vi "CSV Log Loop.vi"(8 "error in (no error)":errorcluster, 11 "Message Queues":T65) -> (0 "error out":errorcluster)   [LabVIEW 2018, in "CSV Log.lvlib"]
uses:
  CSV Log.lvlib
  Main/Main Queue Cluster.ctl
  support/Message Queue/Message Cluster.ctl
  Drag and Drop/State Cluster.ctl
  Drag and Drop/Thumbnail Cluster.ctl
  Drag and Drop/Object Cluster.ctl
  <vilib>/Utility/miscctls.llb/LVRectTypeDef.ctl
  Drag and Drop/Object Type Enum.ctl
  <vilib>/Utility/miscctls.llb/LVPositionTypeDef.ctl
  Config Module/Controls/Main Config Cluster.ctl
  OPC/OPC Module Config.ctl
  Scale Module Folder/Measure Instrument/State Enum.ctl
  <vilib>/Utility/miscctls.llb/LVPoint32TypeDef.ctl
  OPC/OPC Settings.ctl
  OPC/Variable Data Cluster.ctl
  <vilib>/OPCUA/controls/NodeId.ctl
  <vilib>/OPCUA/controls/OPC UA StatusCode.ctl
  <vilib>/OPCUA/controls/Subscription ID.ctl
  <vilib>/OPCUA/controls/OPC UA Client Refnum.ctl
  <vilib>/OPCUA/controls/Subscription Data Change.ctl
  <vilib>/OPCUA/controls/Data Type.ctl
  Feed Module/Controls/Feed Module Config Cluster.ctl
  Feed Module/Controls/Feed Module Settings Cluster.ctl
  Ismatec ISM 831C/Controls/Ismatech Settings Cluster.ctl
  Masterflex 7550-30/Controls/Settings Cluster.ctl
  Mettler Toledo/Controls/Settings Cluster.ctl
  Bronkhorst M13 Flow Meter/Settings Cluster.ctl
  Measure Instrument/PID 2 Parameters Cluster.ctl
  Measure Instrument/PID Input Enum.ctl
  Measure Instrument/PID 2 Output Enum.ctl
  Tacmina QI/Tacmina QI DAQ Setting.ctl
  KNF Pump/Settings Cluster plus SIMDOS.ctl
  ASIA Pump/Pump Settings.ctl
  VICI M50 Party Mode/Settings Cluster.ctl
  FLOM Pump/Settings Cluster.ctl
  SSI PR Class/SSI PR or LD Settings Cluster.ctl
  Masterflex 75211/Masterflex 75211 DAQ Setting.ctl
  SSI PR Class/SSI P40 Settings Cluster.ctl
  TT Module/Controls/TT Module Config Cluster.ctl
  Tag VIs/Numeric Alarm Settings Cluster.ctl
  Acquisition/Hardware Configuration.ctl
  Acquisition/Task Cluster.ctl
  PT Module/Controls/PT Module Config Cluster.ctl
  Scale Module Folder/Feed Module/Controls/Scale Module Config Cluster.ctl
  Scale Module Folder/Feed Module/Controls/Scale Module Settings Cluster.ctl
  Pump Module Folder/Pump Module Config Cluster.ctl
  Pump Module Folder/Pump Module Settings Cluster.ctl
  LabJack Module/Controls/U3 Module Config Cluster.ctl
  Decoration Module/Decoration Module Config Cluster.ctl
  Flow Module Folder/Feed Module/Controls/Flow Module Config Cluster.ctl
  Flow Module Folder/Feed Module/Controls/Flow Module Settings Cluster.ctl
  TCU Module/TCU Module Folder/TCU Module Config Cluster.ctl
  TCU Module/TCU Module Folder/TCU Module Settings Cluster.ctl
  TCU Module/TCU Module Folder/Measure Instrument/Output Devices.ctl
  Huber TCU/Huber Settings.ctl
  Lauda Integral XT-150 TCU/Lauda Settings.ctl
  Julabo Type 1 TCU/Julabo Type 1 TCU Folder/Julabo FP-50 Settings.ctl
  Huber Unistat 410 TCU/Huber Unistat 410 RS485 Settings.ctl
  D-O Module Folder/Not Sure Where this is Used.ctl
  Sequencing/Squence Control.ctl
  D-O Module Folder/D-O Module Config Cluster.ctl
  D-O Module Folder/Valve Clusters.ctl
  D-O Module Folder/D-O Module Settings Cluster.ctl
  D-O Module Folder/D-O Device Settings Cluster.ctl
  VICI Electronic Actuator/VICI Electronic Actuator Settings.ctl
  Pressure Regulator Control Module/Pressure Regulator/Controls/4-20mA Module Config Cluster.ctl
  Pressure Regulator Control Module/Pressure Regulator/Controls/4-20mA Module Settings Cluster.ctl
  Pressure Transmitter/Pressure Transmitter Device Settings.ctl
  Pressure Reg Module/Pressure Regulator Device Settings.ctl
  CSV Log State Cluster.ctl
  support/Message Queue/Enqueue Message (Single).vi
  support/Message Queue/Message Queue.lvlib
  support/Command Log VIs/Command Logging.lvlib
  TT Module/TT Module.lvlib
  Ismatec ISM 831C/Ismatec ISM 831C.lvlib
  Masterflex 7550-30/Masterflex 7550-30.lvlib
  Mettler Toledo/Mettler Toledo.lvlib
  Bronkhorst M13 Flow Meter/Bronkhorst M13 Flow Meter.lvlib
  Tacmina QI/Tacmina QI.lvlib
  KNF Pump/KNF SIMDOS.lvlib
  ASIA Pump.lvlib
  VICI M50 Party Mode/VICI M6 M50 Party Mode.lvlib
  Feed Module/Feed Module.lvlib
  DAQ/DAQ.lvlib
  PT Module/PT Module.lvlib
  Scale Module Folder/Scale Module.lvlib
  Pump Module Folder/Pump Module.lvlib
  LabJack Module/U3 Module.lvlib
  Flow Module Folder/Flow Module.lvlib
  Huber TCU/Huber Ministat 230 TCU.lvlib
  Lauda Integral XT-150 TCU/Lauda TCU.lvlib
  Julabo Type 1 TCU/Julabo Type 1 TCU Folder/Julabo Type FP-50 TCU.lvlib
  TCU Module/TCU Module Folder/TCU Module.lvlib
  Sequencing/Sequencing Library.lvlib
  D-O Module Folder/D-O Module.lvlib
  Config Module/Config Module.lvlib
  Drag and Drop/Drag and Drop.lvlib
  Pressure Transmitter/Pressure Transmitter Library.lvlib
  Pressure Regulator Control Module/Pressure Regulator/4-20mA Module.lvlib
  Pressure Reg Module/Pressure Regulator Library.lvlib
  FLOM Pump/FLOM Pump.lvlib
  SSI PR Class/SSI PR or LD Pump.lvlib
  OPC/OPC UA.lvlib
  Scale Module Folder/Measure Instrument/Scale Module Engine.lvlib
  D-O Module Folder/DIO Valve/VICI Electronic Actuator.lvlib
  Masterflex 75211/Masterflex 75211.lvlib
  SSI PR Class/SSI P40 Pump.lvlib
  Huber Unistat 410 TCU/Huber Unistat 410 TCU.lvlib
panel:
  in  "?":T1 {"Main Config"."PR Module Configs"."Settings"."PID 2 Parameters"."output range"."output low" format="%.2f"; "Main Config"."PR Module Configs"."Settings"."PID 2 Parameters"."output range"."output high" min=0.0 max=100.0 format="%.2f"; "Main Config"."PR Module Configs"."Settings"."PID 2 Parameters"."PID gains"."derivative time (Td, min)" format="%.3f"; "Main Config"."PR Module Configs"."Settings"."PID 2 Parameters"."PID gains"."integral time (Ti, min)" format="%.3f"; "Main Config"."PR Module Configs"."Settings"."PID 2 Parameters"."PID gains"."proportional gain (Kc)" format="%.3f"; "Main Config"."Steps"."Control" items=["Pump %", "Setpoint"]; "Main Config"."TCU Module Configs"."Settings"."Huber Unistat 410 Settings"."Address" min=0 max=99 format="%02.0f"; "Main Config"."TCU Module Configs"."Settings"."Julabo FP-50 Settings"."Pump Power" min=0 max=8 step=1; "Main Config"."TCU Module Configs"."Settings"."Lauda Settings"."Pump Power" min=0 max=8 step=1; "Main Config"."Pump Module Configs"."Settings"."ASIA Pump C"."channel" min=0 max=1 step=1; "Main Config"."Pump Module Configs"."Settings"."Masterflex"."Pump Number" min=1.0 max=20.0 step=1.0; "Main Config"."Pump Module Configs"."Settings"."Ismatech"."Pump Number" min=1.0 max=20.0 step=1.0; "Main Config"."Feed Module Configs"."Settings"."output range"."output low" min=0.0 max=100.0 format="%.2f"; "Main Config"."Feed Module Configs"."Settings"."output range"."output high" format="%.2f"; "Main Config"."Feed Module Configs"."Settings"."PID 2 Parameters"."PID gains"."derivative time (Td, min)" format="%.3f"; "Main Config"."Feed Module Configs"."Settings"."PID 2 Parameters"."PID gains"."integral time (Ti, min)" format="%.3f"; "Main Config"."Feed Module Configs"."Settings"."PID 2 Parameters"."PID gains"."proportional gain (Kc)" format="%.3f"; "Main Config"."Feed Module Configs"."Settings"."ASIA Pump C"."channel" min=0 max=1 step=1; "Main Config"."Feed Module Configs"."Settings"."Ismatech"."Pump Number" min=1.0 max=20.0 step=1.0; "Main Config"."Feed Module Configs"."Settings"."Masterflex"."Pump Number" min=1.0 max=20.0 step=1.0}
  in  "?":T1 {"Main Config"."PR Module Configs"."Settings"."PID 2 Parameters"."output range"."output low" format="%.2f"; "Main Config"."PR Module Configs"."Settings"."PID 2 Parameters"."output range"."output high" min=0.0 max=100.0 format="%.2f"; "Main Config"."PR Module Configs"."Settings"."PID 2 Parameters"."PID gains"."derivative time (Td, min)" format="%.3f"; "Main Config"."PR Module Configs"."Settings"."PID 2 Parameters"."PID gains"."integral time (Ti, min)" format="%.3f"; "Main Config"."PR Module Configs"."Settings"."PID 2 Parameters"."PID gains"."proportional gain (Kc)" format="%.3f"; "Main Config"."Steps"."Control" items=["Pump %", "Setpoint"]; "Main Config"."TCU Module Configs"."Settings"."Huber Unistat 410 Settings"."Address" min=0 max=99 format="%02.0f"; "Main Config"."TCU Module Configs"."Settings"."Julabo FP-50 Settings"."Pump Power" min=0 max=8 step=1; "Main Config"."TCU Module Configs"."Settings"."Lauda Settings"."Pump Power" min=0 max=8 step=1; "Main Config"."Pump Module Configs"."Settings"."ASIA Pump C"."channel" min=0 max=1 step=1; "Main Config"."Pump Module Configs"."Settings"."Masterflex"."Pump Number" min=1.0 max=20.0 step=1.0; "Main Config"."Pump Module Configs"."Settings"."Ismatech"."Pump Number" min=1.0 max=20.0 step=1.0; "Main Config"."Feed Module Configs"."Settings"."output range"."output low" min=0.0 max=100.0 format="%.2f"; "Main Config"."Feed Module Configs"."Settings"."output range"."output high" format="%.2f"; "Main Config"."Feed Module Configs"."Settings"."PID 2 Parameters"."PID gains"."derivative time (Td, min)" format="%.3f"; "Main Config"."Feed Module Configs"."Settings"."PID 2 Parameters"."PID gains"."integral time (Ti, min)" format="%.3f"; "Main Config"."Feed Module Configs"."Settings"."PID 2 Parameters"."PID gains"."proportional gain (Kc)" format="%.3f"; "Main Config"."Feed Module Configs"."Settings"."ASIA Pump C"."channel" min=0 max=1 step=1; "Main Config"."Feed Module Configs"."Settings"."Ismatech"."Pump Number" min=1.0 max=20.0 step=1.0; "Main Config"."Feed Module Configs"."Settings"."Masterflex"."Pump Number" min=1.0 max=20.0 step=1.0}
  # "Instrument Settings"
  # "Instrument Settings"
  # "Output Instruments"
  # "Flow Meter Settings"
  # "Output Instruments"
  # "Scale Settings"
  # "Output Instruments"
  # "Input Instruments"
  # "Instrument Settings"
  # "Instrument Settings"
  # "Output Instruments"
  # "Flow Meter Settings"
  # "Output Instruments"
  # "Scale Settings"
  # "Output Instruments"
  # "Input Instruments"
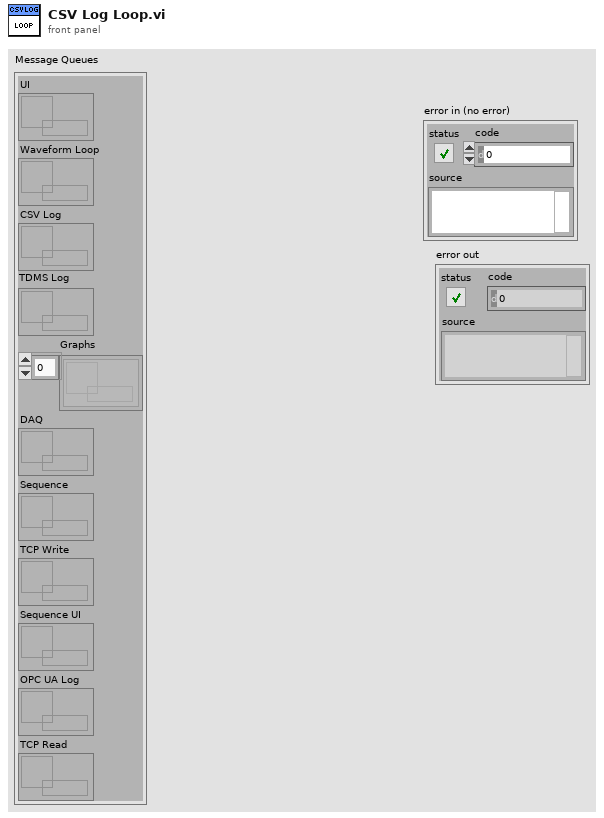
[diagram p1: front panel]
types:
  T1 = typedef "Drag and Drop.lvlib/State Cluster.ctl" = cluster{"VI refs":refnum<vi>[], "Queues":refnum<queue>[], "[Thumbnails]":T2[], "Drag Object Idx":i32, "[Objects]":T3[], "Active Object":i32, "Drop Offset":T6, "Process Name":string, "Main Config":T7, "Campaign Filepath":path, "Config Changed?":bool}
  T2 = typedef "Thumbnail Cluster.ctl" = cluster{"Path":path, "Rectangle":cluster{"left":i16, "top":i16, "right":i16, "bottom":i16}}
  T3 = typedef "Object Cluster.ctl" = cluster{"BMP Path":path, "Anchor Position":cluster{"X":i32, "Y":i32}, "Hot Spot":T4, "Type":T5, "Parameters":variant}
  T4 = typedef "LVRectTypeDef.ctl" = cluster{"Left":i16, "Top":i16, "Right":i16, "Bottom":i16}
  T5 = typedef "Object Type Enum.ctl" = enum16{"Icon", "Line", "Text", "Feed Module"}
  T6 = typedef "LVPositionTypeDef.ctl" = cluster{"Left":i32, "Top":i32}
  T7 = typedef "Config Module.lvlib/Main Config Cluster.ctl" = cluster{"Notebook":string, "Page":string, "OPC Module Configs":T8[], "Feed Module Configs":T17[], "Log File Path":path, "TT Module Configs":T34[], "DAQ Config":T36, "PT Module Configs":T38[], "Scale Module Configs":T39[], "Pump Module Configs":T41[], "U3 Module Configs":T43[], "Decoration Module Configs":T44[], "Flow Module Configs":T45[], "TCU Module Configs":T47[], "Steps":T54, "Abort":bool, "DO Module Configs":T56[], "PR Module Configs":T61[], "Cycle Period":dbl}
  T8 = typedef "OPC UA.lvlib/OPC Module Config.ctl" = cluster{"State":T9, "GUID":string, "Drop Coords":T10, "Configuration":T11, "First Iteration":bool, "Data":cluster{"Object Name":string, "Variable Array":T12[]}[], "Process Name":string, "Load Count":i32, "Log Started":bool, "subscription ID out":T15, "OPC UA client refnum out":T16, "Event Registration Refnum":refnum<event-registration>, "Start Time":timestamp, "Current Time":timestamp}
  T9 = typedef "Scale Module.lvlib/Scale Module Engine.lvlib/State Enum.ctl" = enum16{"Measuring", "Idle"}
  T10 = typedef "LVPoint32TypeDef.ctl" = cluster{"Horizontal":i32, "Vertical":i32}
  T11 = typedef "OPC UA.lvlib/OPC Settings.ctl" = cluster{"Cycle Period":dbl, "server endpoint URL":string, "security policy":cluster{"message mode":enum16{"None", "Sign", "Sign and Encrypt"}, "security":enum16{"Basic256", "Basic128Rsa15"}}, "Trust Any Server":bool}
  T12 = typedef "OPC UA.lvlib/Variable Data Cluster.ctl" = cluster{"node ID":T13, "browse name":string, "status":T14, "timestamp":timestamp, "value ":variant}
  T13 = typedef "NodeId.ctl" = string
  T14 = typedef "OPC UA StatusCode.ctl" = u32
  T15 = typedef "Subscription ID.ctl" = u32
  T16 = typedef "OPC UA Client Refnum.ctl" = refnum<k21>
  T17 = typedef "Feed Module.lvlib/Feed Module Config Cluster.ctl" = cluster{"GUID":string, "Drop Coords":T10, "Process Name":string, "Queue Name":string, "Settings":T18, "Settings Load Count":i32, "OP Load Count":i32}
  T18 = typedef "Feed Module.lvlib/Feed Module Settings Cluster.ctl" = cluster{"Cycle Period":dbl, "Ismatech":T19, "Masterflex":T20, "Mettler":T21, "Bronkhorst M13 Flow Meter":T22, "PID 2 Parameters":T23, "Manual Entry":dbl, "Auto?":bool, "output range":cluster{"output high":dbl, "output low":dbl}, "Bronkhorst M14":T21, "Tacmina Settings":T26, "KNF SIMDOS Settings":T27, "ASIA Pump C":T28, "VICI Settings":T29, "FLOM Settings":T30, "SSI PR/LD Settings":T31, "Masterflex 75211 Settings":T32, "SSI P40 Settings":T33}
  T19 = typedef "Ismatec ISM 831C.lvlib/Ismatech Settings Cluster.ctl" = cluster{"VISA resource name":refnum<visa-resource-name>, "Simulated?":bool, "Pump Number":dbl, "Reverse?":bool}
  T20 = typedef "Masterflex 7550-30.lvlib/Settings Cluster.ctl" = cluster{"VISA resource name":refnum<visa-resource-name>, "Simulated?":bool, "Pump Number":dbl, "Reverse?":bool}
  T21 = typedef "Mettler Toledo.lvlib/Settings Cluster.ctl" = cluster{"VISA resource name":refnum<visa-resource-name>, "Simulated?":bool}
  T22 = typedef "Bronkhorst M13 Flow Meter.lvlib/Settings Cluster.ctl" = cluster{"VISA resource name":refnum<visa-resource-name>, "Simulated?":bool}
  T23 = typedef "PID 2 Parameters Cluster.ctl" = cluster{"Input Device":T24, "Output Device":T25, "Setpoint":dbl, "PID gains":cluster{"proportional gain (Kc)":dbl, "integral time (Ti, min)":dbl, "derivative time (Td, min)":dbl}}
  T24 = typedef "PID Input Enum.ctl" = enum16{"Default", "Bronkhorst M13", "Bronkhorst M14", "Scale Rate of Change"}
  T25 = typedef "PID 2 Output Enum.ctl" = enum16{"Default", "Ismatec ISM 831C", "Masterflex 7550-30", "VICI", "Tacmina QI", "KNF SIMDOS", "ASIA Type C", "FLOM UI-22-11", "SSI PR/LD", "SSI P40", "Masterflex 75211-70"}
  T26 = typedef "Tacmina QI.lvlib/Tacmina QI DAQ Setting.ctl" = cluster{"Analog DAQ Task":refnum<k21>, "Digital DAQ Task":refnum<k21>}
  T27 = typedef "KNF SIMDOS.lvlib/Settings Cluster plus SIMDOS.ctl" = cluster{"VISA resource name":refnum<visa-resource-name>, "Simulated?":bool}
  T28 = typedef "ASIA Pump.lvlib/Pump Settings.ctl" = cluster{"ASIA Pump #":i32, "channel":i32, "Simulated":bool}
  T29 = typedef "VICI M6 M50 Party Mode.lvlib/Settings Cluster.ctl" = cluster{"VISA resource name":refnum<visa-resource-name>, "Simulated?":bool, "Pump Letter":string, "Reverse?":bool}
  T30 = typedef "FLOM Pump.lvlib/Settings Cluster.ctl" = cluster{"VISA resource name":refnum<visa-resource-name>, "Simulated?":bool, "Pump Number":dbl}
  T31 = typedef "SSI PR or LD Pump.lvlib/SSI PR or LD Settings Cluster.ctl" = cluster{"VISA resource name":refnum<visa-resource-name>, "Simulated?":bool}
  T32 = typedef "Masterflex 75211.lvlib/Masterflex 75211 DAQ Setting.ctl" = cluster{"Analog DAQ Task":refnum<k21>, "Digital DAQ Task":refnum<k21>}
  T33 = typedef "SSI P40 Pump.lvlib/SSI P40 Settings Cluster.ctl" = cluster{"VISA resource name":refnum<visa-resource-name>, "Simulated?":bool}
  T34 = typedef "TT Module.lvlib/TT Module Config Cluster.ctl" = cluster{"GUID":string, "Drop Coords":T10, "Input Channel Tag Name ":string, "Process Name":string, "Queue Name":string, "Input Channel Numeric Alarm Settings":T35[]}
  T35 = typedef "Numeric Alarm Settings Cluster.ctl" = cluster{"enable? (F)":bool, "name":string, "alarm type":enum16{"HI_HI", "HI", "LO", "LO_LO"}, "level/change":dbl, "deadband/time":dbl, "alarm delay":dbl, "priority":u32, "ack type":enum16{"Auto", "User", "None", "Each Occurrence"}, "area":string, "description":string, "log? (T)":bool}
  T36 = typedef "DAQ.lvlib/Hardware Configuration.ctl" = cluster{"Tasks":T37[]}
  T37 = typedef "Task Cluster.ctl" = cluster{"DAQmx Task":refnum<k21>, "Read-Write Radio":enum32{"Read", "Write"}}
  T38 = typedef "PT Module.lvlib/PT Module Config Cluster.ctl" = cluster{"GUID":string, "Drop Coords":T10, "Input Channel Tag Name ":string, "Process Name":string, "Queue Name":string, "Input Channel Numeric Alarm Settings":T35[]}
  T39 = typedef "Scale Module.lvlib/Scale Module Config Cluster.ctl" = cluster{"GUID":string, "Drop Coords":T10, "Process Name":string, "Queue Name":string, "Settings":T40, "Load Count":i32}
  T40 = typedef "Scale Module.lvlib/Scale Module Settings Cluster.ctl" = cluster{"Cycle Period":dbl, "Mettler":T21, "Scale Type":string}
  T41 = typedef "Pump Module.lvlib/Pump Module Config Cluster.ctl" = cluster{"GUID":string, "Drop Coords":T10, "Process Name":string, "Queue Name":string, "Settings":T42, "Load Count":i32}
  T42 = typedef "Pump Module.lvlib/Pump Module Settings Cluster.ctl" = cluster{"Cycle Period":dbl, "Manual Entry":dbl, "Output Device":T25, "Ismatech":T19, "Masterflex":T20, "VICI Settings":T29, "Tacmina Settings":T26, "KNF SIMDOS Settings":T27, "ASIA Pump C":T28, "FLOM Settings":T30, "SSI PR/LD Settings":T31, "SSI P40 Settings":T31, "Masterflex 75211 Settings":T32, "Pump Calibration File":path, "Calibration Slope":dbl, "Calibration Y Intercept":dbl, "Pump Cal Enum":u16}
  T43 = typedef "U3 Module.lvlib/U3 Module Config Cluster.ctl" = cluster{"GUID":string, "Drop Coords":T10, "AI Channel Number":enum16{"Default", "AI0", "AI1", "AI2", "AI3", "AI4", "AI5", "AI6", "AI7"}, "Process Name":string, "Queue Name":string, "Input Channel Numeric Alarm Settings":T35[]}
  T44 = typedef "Decoration Module Config Cluster.ctl" = cluster{"GUID":string, "Drop Coords":T10, "Decoration Filepath":path}
  T45 = typedef "Flow Module.lvlib/Flow Module Config Cluster.ctl" = cluster{"GUID":string, "Drop Coords":T10, "Process Name":string, "Queue Name":string, "Settings":T46, "Load Count":i32}
  T46 = typedef "Flow Module.lvlib/Flow Module Settings Cluster.ctl" = cluster{"Cycle Period":dbl, "Bronkhorst M13":T21, "Flow Meter Type":string, "Bronkhorst M14":T21}
  T47 = typedef "TCU Module.lvlib/TCU Module Config Cluster.ctl" = cluster{"GUID":string, "Drop Coords":T10, "Process Name":string, "Queue Name":string, "Settings":T48, "Load Count":i32, "Power Level Changed":bool}
  T48 = typedef "TCU Module.lvlib/TCU Module Settings Cluster.ctl" = cluster{"Cycle Period":dbl, "Setpoint Entry":dbl, "Output Device":T49, "Huber Ministat 230 Settings":T50, "Lauda Settings":T51, "Julabo FP-50 Settings":T52, "Internal Control?":bool, "Huber Unistat 410 Settings":T53}
  T49 = typedef "Output Devices.ctl" = enum16{"Default", "Huber Ministat 230", "Huber Unistat 410", "Lauda XT-150", "Julabo FP-50"}
  T50 = typedef "Huber Ministat 230 TCU.lvlib/Huber Settings.ctl" = cluster{"VISA resource name":refnum<visa-resource-name>, "Simulated?":bool}
  T51 = typedef "Lauda TCU.lvlib/Lauda Settings.ctl" = cluster{"VISA resource name":refnum<visa-resource-name>, "Simulated?":bool, "Pump Power":i32}
  T52 = typedef "Julabo Type FP-50 TCU.lvlib/Julabo FP-50 Settings.ctl" = cluster{"VISA resource name":refnum<visa-resource-name>, "Simulated?":bool, "Pump Power":i32}
  T53 = typedef "Huber Unistat 410 TCU.lvlib/Huber Unistat 410 RS485 Settings.ctl" = cluster{"VISA resource name":refnum<visa-resource-name>, "Address":i8, "Simulated?":bool}
  T54 = typedef "Not Sure Where this is Used.ctl" = T55[]
  T55 = typedef "Sequencing Library.lvlib/Squence Control.ctl" = cluster{"Module":string, "Control":u16, "Value":dbl, "Wait (sec)":dbl}
  T56 = typedef "D-O Module.lvlib/D-O Module Config Cluster.ctl" = cluster{"GUID":string, "Drop Coords":T10, "Process Name":string, "Queue Name":string, "Settings":T57, "Load Count":i32}
  T57 = typedef "D-O Module.lvlib/Valve Clusters.ctl" = cluster{"Valve Settings":T58, "Valve Type":enum16{"Default", "Digital Output Valve", "VICI Electronic Actuator"}, "Time On (Sec)":dbl, "Time Off (Sec)":dbl, "Run?":bool}
  T58 = typedef "D-O Module.lvlib/D-O Module Settings Cluster.ctl" = cluster{"D-O Settings":T59, "VICI Electronic Actuator":T60}
  T59 = typedef "D-O Module.lvlib/D-O Device Settings Cluster.ctl" = cluster{"DAQmx Task Name":refnum<k21>, "Output Channel":u16, "Output Channel Names":string[]}
  T60 = typedef "VICI Electronic Actuator.lvlib/VICI Electronic Actuator Settings.ctl" = cluster{"VISA resource name":refnum<visa-resource-name>, "Mode":enum16{"Two Positions With Stops", "Two Positions Without Stops", "Mutiposition"}, "Simulated":bool}
  T61 = typedef "4-20mA Module.lvlib/4-20mA Module Config Cluster.ctl" = cluster{"GUID":string, "Drop Coords":T10, "Process Name":string, "Queue Name":string, "Settings":T62, "Settings Load Count":i32}
  T62 = typedef "4-20mA Module.lvlib/4-20mA Module Settings Cluster.ctl" = cluster{"Cycle Period":dbl, "PID 2 Parameters":cluster{"Input Device":enum16{"Default", "4-20mA"}, "Output Device":enum16{"Default", "Equilibar Pressure Reg", "Flow Regulator"}, "Setpoint":dbl, "PID gains":cluster{"proportional gain (Kc)":dbl, "integral time (Ti, min)":dbl, "derivative time (Td, min)":dbl}, "output range":cluster{"output low":dbl, "output high":dbl}}, "Manual Entry":dbl, "Auto?":bool, "4-20mA Input Settings":T63, "4-20mA Out Settings":T64, "Input Channel Tag Name ":string}
  T63 = typedef "Pressure Transmitter Library.lvlib/Pressure Transmitter Device Settings.ctl" = cluster{"Input Channel ":u16}
  T64 = typedef "Pressure Regulator Library.lvlib/Pressure Regulator Device Settings.ctl" = cluster{"Output DAQ Task":refnum<k21>}
  T65 = typedef "Main Queue Cluster.ctl" = cluster{"UI":refnum<queue>, "Waveform Loop":refnum<queue>, "CSV Log":refnum<queue>, "TDMS Log":refnum<queue>, "Graphs":refnum<queue>[], "DAQ":refnum<queue>, "Sequence":refnum<queue>, "TCP Write":refnum<queue>, "Sequence UI":refnum<queue>, "OPC UA Log":refnum<queue>, "TCP Read":refnum<queue>}
  T66 = typedef "CSV Log.lvlib/CSV Log State Cluster.ctl" = cluster{"CSV log path":path, "CSV refnum":refnum<file>, "Have written headers?":bool, "Notebook":string}
  T67 = enum16{"open", "replace", "create", "open or create", "replace or create", "replace or create with confirmation"}
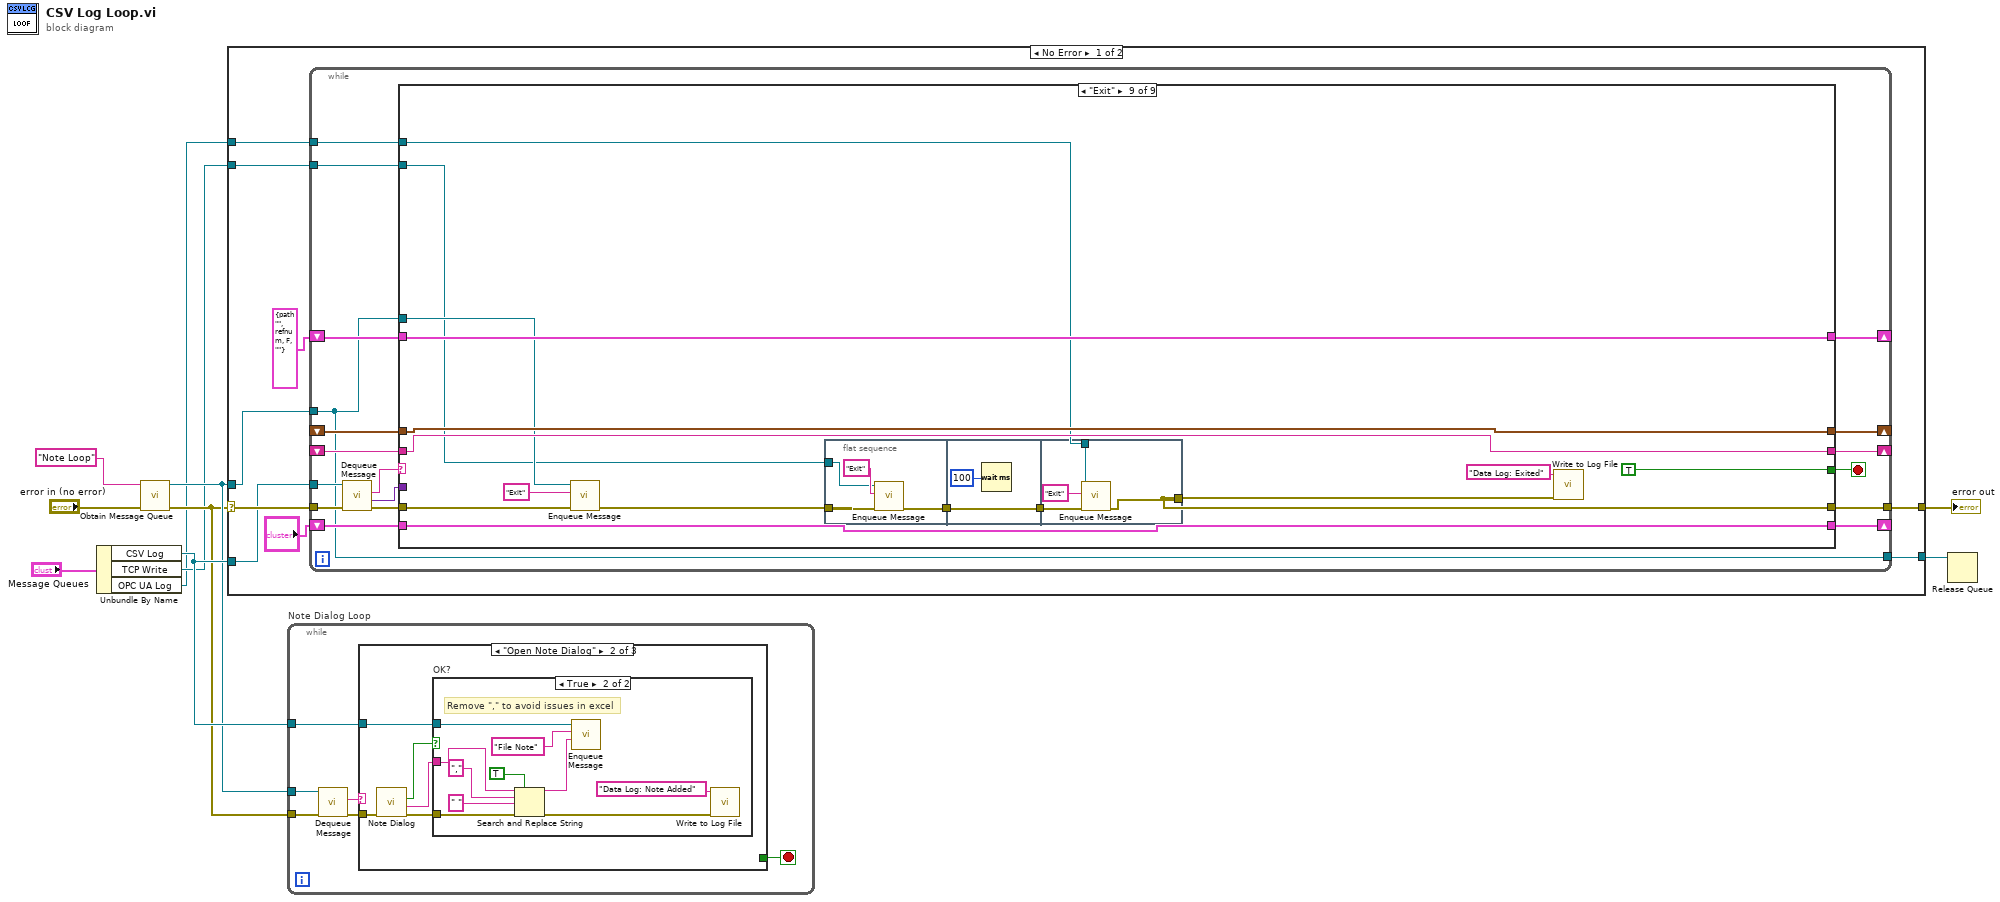
[diagram p0: block diagram]
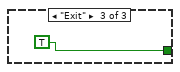
[diagram p4: hidden frame]
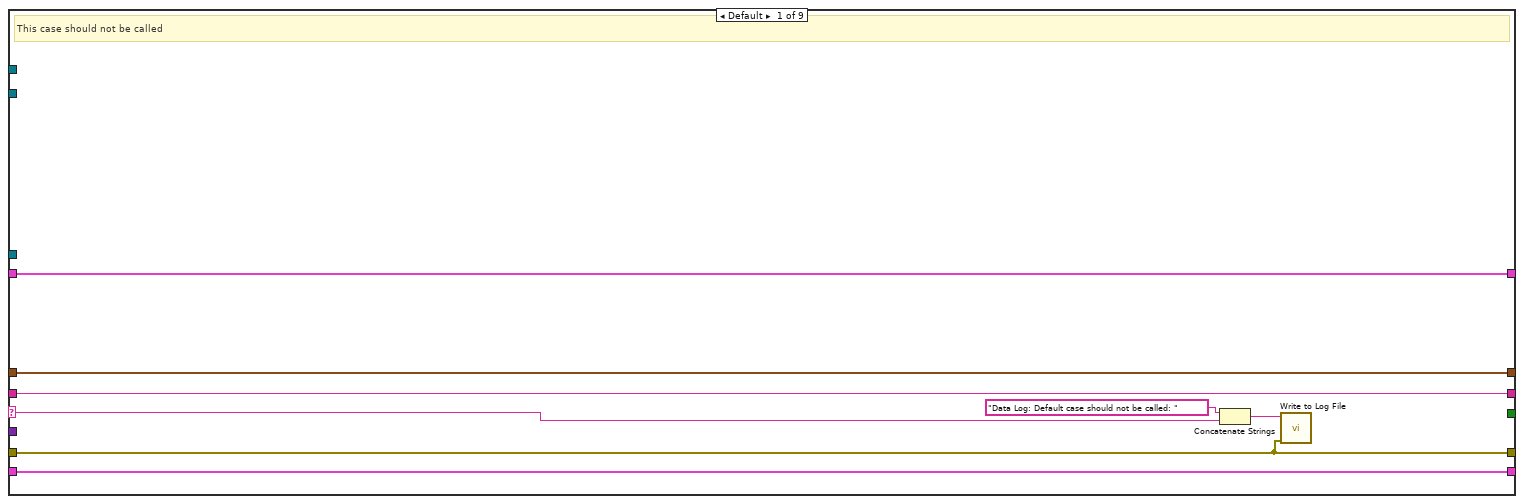
[diagram p5: hidden frame]
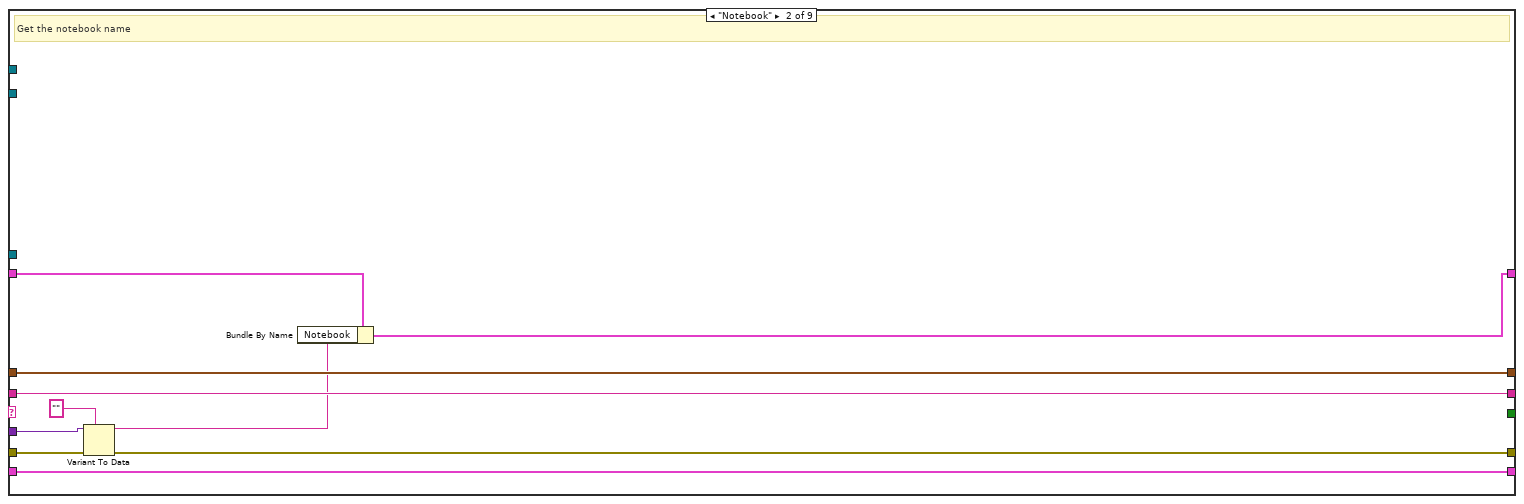
[diagram p6: hidden frame]
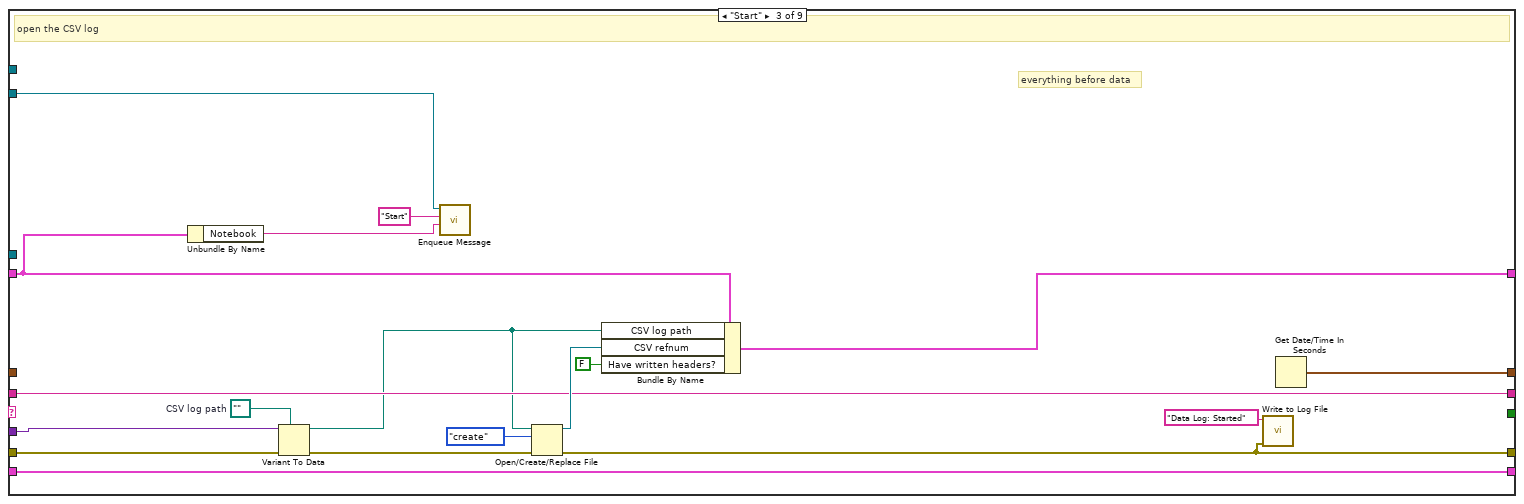
[diagram p7: hidden frame]
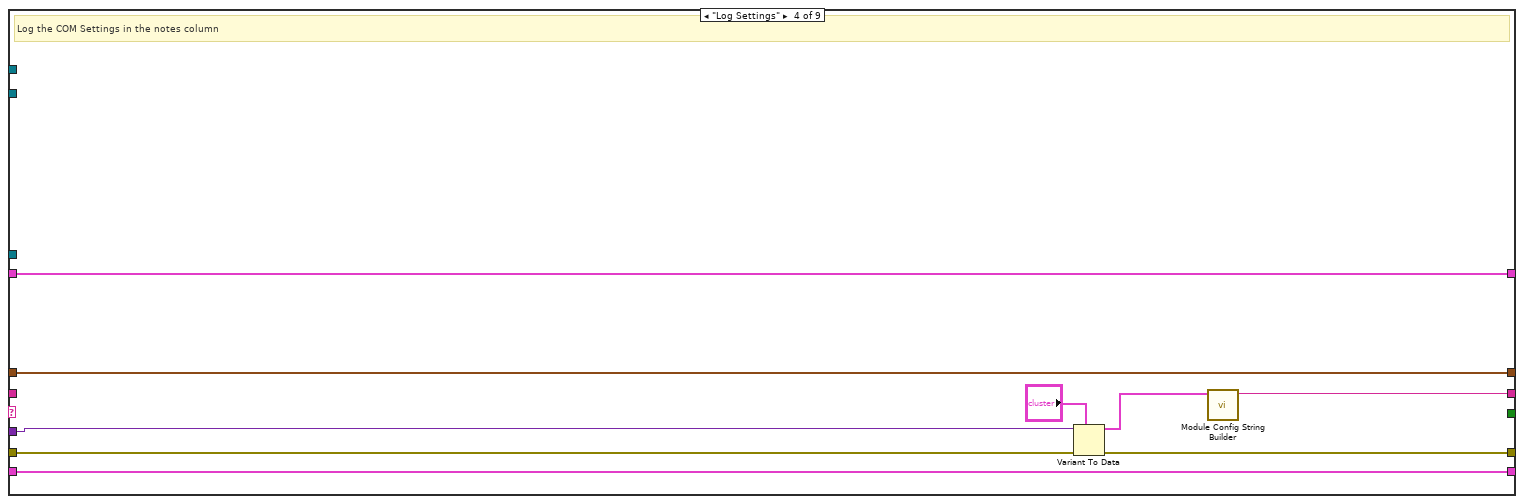
[diagram p8: hidden frame]
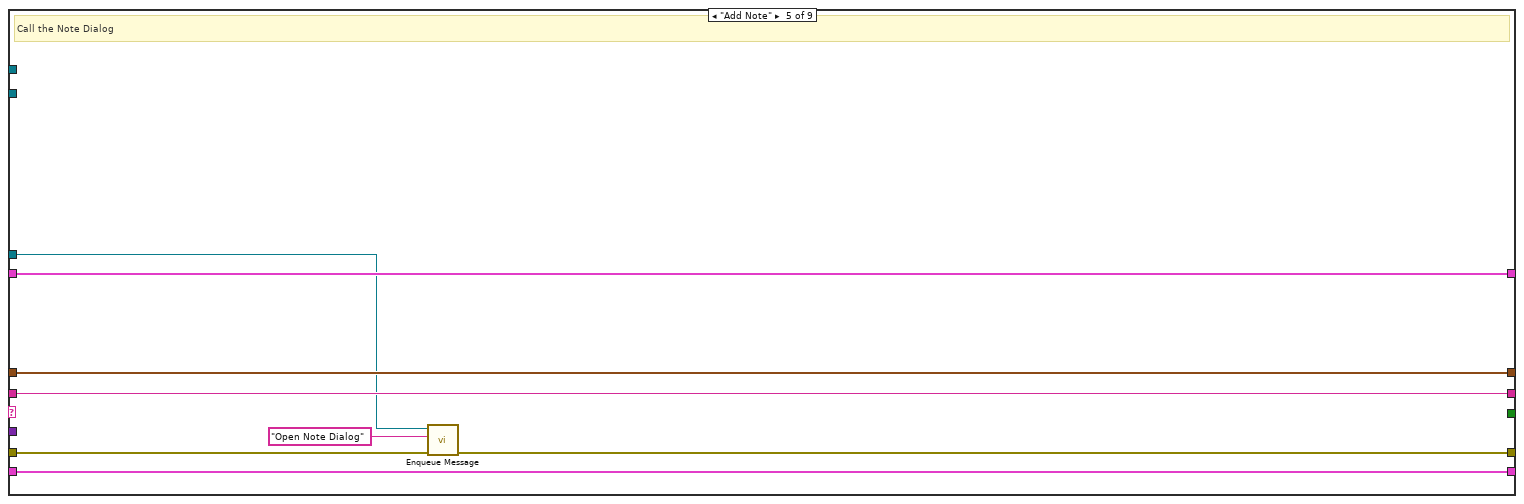
[diagram p9: hidden frame]
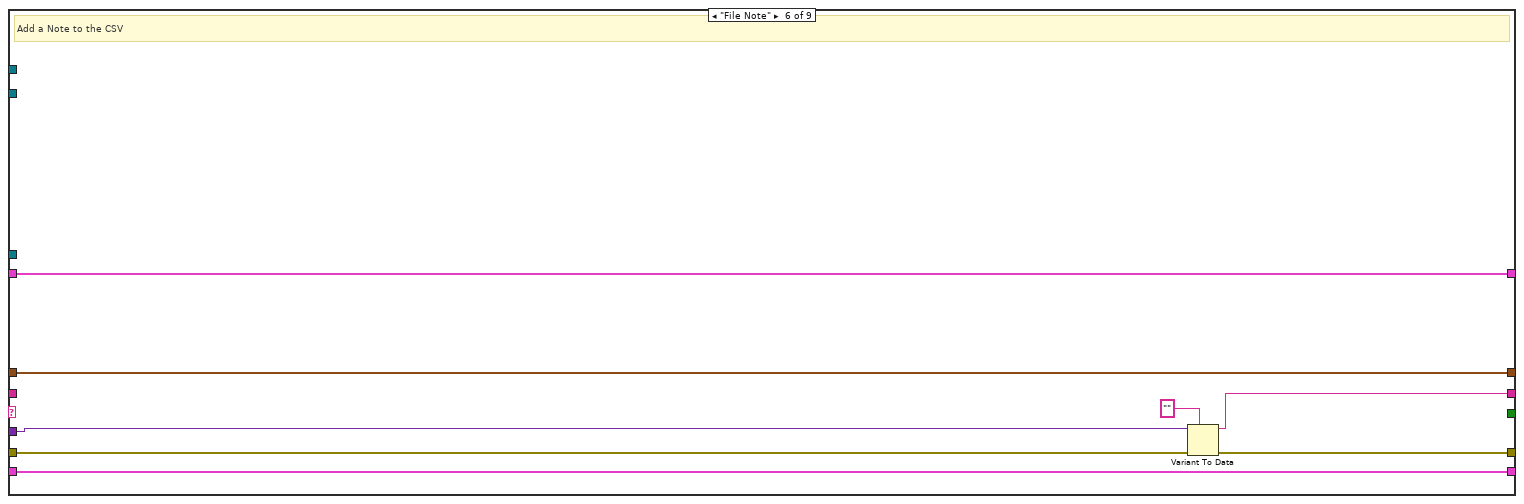
[diagram p10: hidden frame]
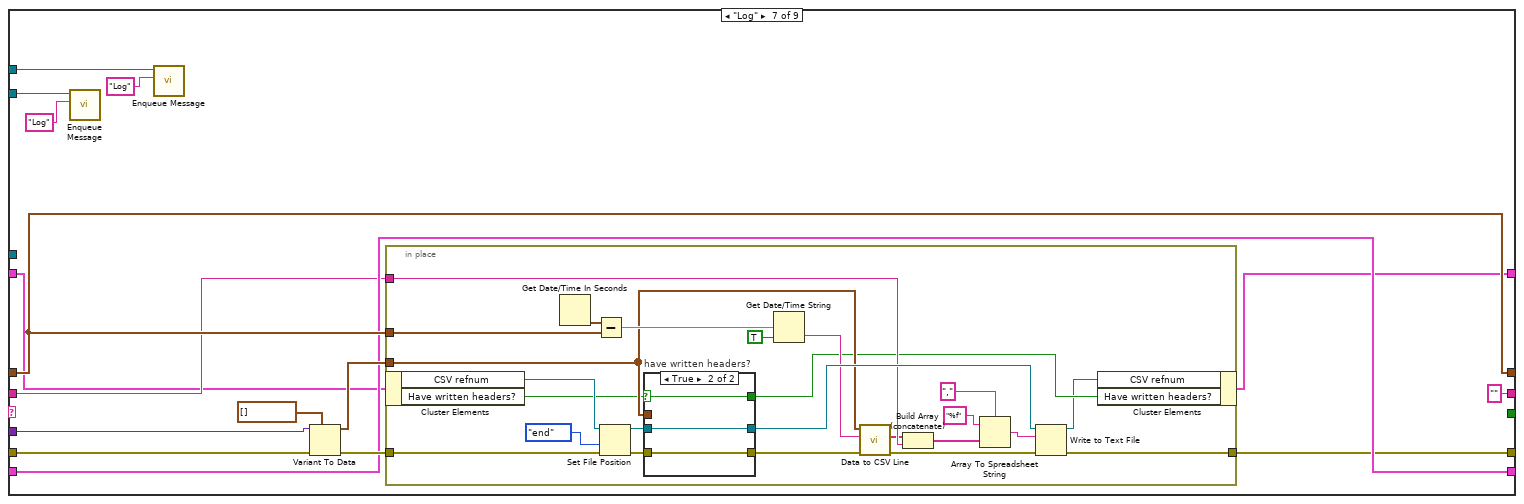
[diagram p11: hidden frame]
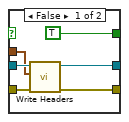
[diagram p12: hidden frame]
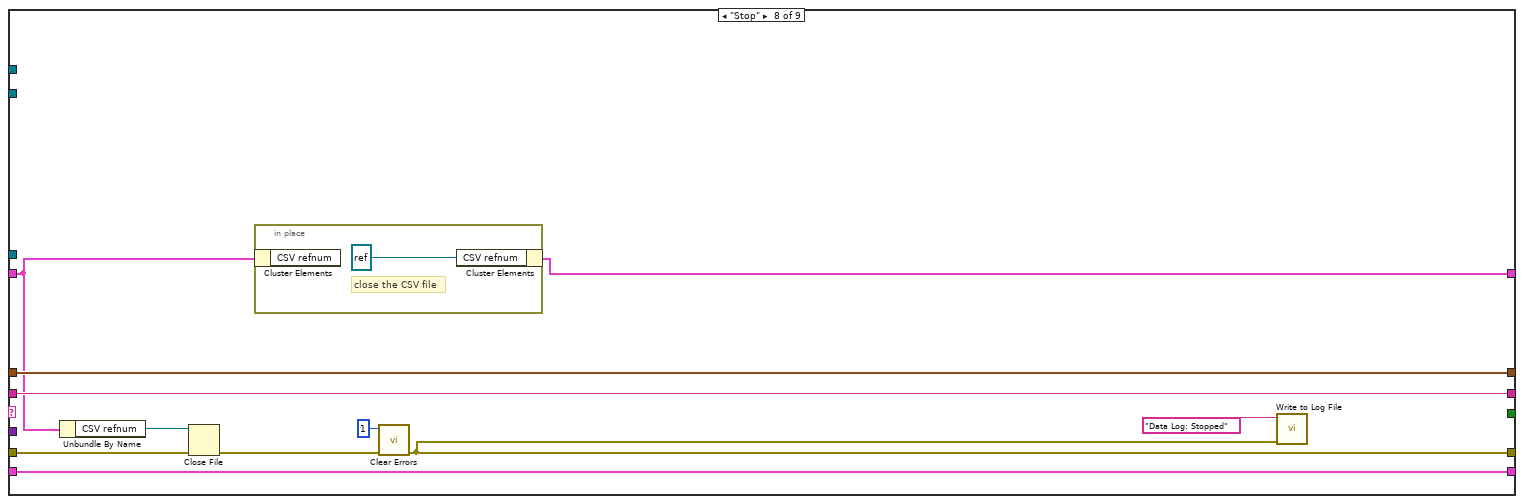
[diagram p13: hidden frame]
diagram:
  n1 = Unbundle By Name("Message Queues") -> ("CSV Log"=w8:refnum<queue>, "TCP Write"=w3:refnum<queue>, "OPC UA Log"=w2:refnum<queue>)
  n2 = call "Obtain Message Queue.vi"("error in (no error)"="error in (no error)", "name (unnamed)"="Note Loop") -> ("error out"=w4:errorcluster, "Message Queue"=w5:refnum<queue>)  [unwired: 8 in]
  n3 = case shown="No Error" w4 {
    selector: w4 -> [w19 w186]
    tunnel: [w15 w186] -> w9
    tunnel: w8 -> [w18 _]
    tunnel: w5 -> [w12 w185]
    tunnel: w3 -> [w14 _]
    tunnel: w2 -> [w13 _]
    tunnel: [w11 w185] -> w1
    frame No Error {
      n4 = while {
        shift-right: [w34] -> _
        shift-left: T66 {"CSV log path"=path "", "CSV refnum"=refnum, "Have written headers?"=FALSE, "Notebook"=""} ("Waveform Loop State") -> [w36]
        tunnel: w19 -> [w31]
        tunnel: [w30] -> w15
        shift-right: [w29] -> _
        shift-left: _ -> [w28]
        shift-right: [w27] -> _
        shift-left: "?" -> [w26]
        shift-right: [w25] -> _
        shift-left: _ -> [w24]
        tunnel: w18 -> [w23]
        tunnel: w12 -> [w20]
        tunnel: w14 -> [w22]
        tunnel: w13 -> [w21]
        tunnel: [w20] -> w11
        stop <- w32 stop-if-true
        n5 = call "Dequeue Message.vi"("error in (no error)"=w31, "Message Queue"=w23) -> ("error out"=w33:errorcluster, "Message Data"=w35:variant, "Message"=w37:string)  [unwired: 6 in, 1 out]
        n6 = case shown="\"Exit\"" w37 {
          selector: w37 -> [w40 _ _ _ _ _ _ _ _]
          tunnel: w36 -> [w45 w47 w57 w78 w89 w97 w99 w149 w174]
          tunnel: w35 -> [_ w52 w73 w82 _ w95 w113 _ _]
          tunnel: [w45 w46 w72 w78 w89 w97 w100 w148 w174] -> w34
          tunnel: w33 -> [w41 w51 w71 w81 w86 w94 w114 w158 w167]
          tunnel: [_ _ _ _ _ _ _ _ TRUE] -> w32
          tunnel: [w41 w50 w62 w76 w85 w91 w105 w151 w160] -> w30
          tunnel: [w44 w55 w66 w77 w88 w96 w111 w156 w172] -> w29
          tunnel: w28 -> [w44 w55 _ w77 w88 w96 w111 w156 w172]
          tunnel: [w43 w54 w65 w80 w90 w98 w108 w155 w171] -> w27
          tunnel: w26 -> [w43 w54 w65 w80 w90 w98 w108 w155 w171]
          tunnel: [w42 w53 w64 w74 w87 w92 "" w154 w170] -> w25
          tunnel: w24 -> [w42 w53 w64 _ w87 _ w107 w154 w170]
          tunnel: w20 -> [_ _ _ _ w84 _ _ _ w168]
          tunnel: w22 -> [_ _ w61 _ _ _ w103 _ w165]
          tunnel: w21 -> [_ _ _ _ _ _ w101 _ w164]
          frame Default {
            # "This case should not be called"
            n7 = Concatenate Strings("Data Log: Default case should not be called: " ("text"), w40) -> (w38:string)
            n8 = call "Write to Log File.vi"("error in"=w41, "text"=w38) -> ()  [unwired: 9 in, 1 out]
          }
          frame "Notebook" {
            # "Get the notebook name"
            n9 = Variant To Data(error in=w51, type="", Variant=w52) -> (data=w48:string, error out=w50:errorcluster)
            n10 = Bundle By Name(cluster=w47, "Notebook"=w48) -> (w46:T66)
          }
          frame "Start" {
            w59 = path ""  # CSV log path
            # "everything before data"
            # "open the CSV log"
            n11 = Unbundle By Name(w57) -> ("Notebook"=w56:string)
            n12 = Variant To Data(error in=w71, type=w59, Variant=w73) -> (data=w58:path, error out=w70:errorcluster)
            n13 = call-poly "Enqueue Message.vi"("Message Data"=w56, "Message"="Start", "Message Queue"=w61) -> ()  [unwired: 7 in, 2 out]
            n14 = Open/Create/Replace File(file path (use dialog)=w58, error in=w70, operation (0:open)=T67."create") -> (refnum out=w68:refnum<file>, error out=w62:errorcluster)  [unwired: 3 in, 1 out]
            n15 = Bundle By Name(cluster=w57, "CSV log path"=w58, "CSV refnum"=w68, "Have written headers?"=FALSE) -> (w72:T66)
            n16 = call "Write to Log File.vi"("error in"=w62, "text"="Data Log: Started") -> ()  [unwired: 9 in, 1 out]
            n17 = Get Date/Time In Seconds() -> (seconds since 1Jan1904=w66:timestamp)
          }
          frame "Log Settings" {
            # "Log the COM Settings in the notes column"
            n18 = Variant To Data(error in=w81, type="?", Variant=w82) -> (data=w75:T1, error out=w76:errorcluster)
            n19 = call "Module Config String Builder.vi"("Cluster"=w75) -> ("Module Configs"=w74:string)  [unwired: 10 in]
          }
          frame "Add Note" {
            # "Call the Note Dialog"
            n20 = call-poly "Enqueue Message.vi"("error in (no error)"=w86, "Message"="Open Note Dialog", "Message Queue"=w84) -> ("error out"=w85:errorcluster)  [unwired: 7 in, 1 out]
          }
          frame "File Note" {
            # "Add a Note to the CSV"
            n21 = Variant To Data(error in=w94, type="", Variant=w95) -> (data=w92:string, error out=w91:errorcluster)
          }
          frame "Log" {
            n22 = call-poly "Enqueue Message.vi"("Message"="Log", "Message Queue"=w103) -> ()  [unwired: 8 in, 2 out]
            n23 = call-poly "Enqueue Message.vi"("Message"="Log", "Message Queue"=w101) -> ()  [unwired: 8 in, 2 out]
            n24 = Variant To Data(error in=w114, type=waveform(dbl)[] [], Variant=w113) -> (data=w110:waveform(dbl)[], error out=w109:errorcluster)
            n25 = in-place {
              in-place-border: w111 -> [w128]
              in-place-border: w110 -> [w127]
              in-place-border: w109 -> [w126]
              in-place-border: w107 -> [w125]
              in-place-border: [w120] -> w105
              n26 = in-place-cluster #1(w99) -> ("CSV refnum"=w118:refnum<file>, "Have written headers?"=w117:bool)
              n27 = Get Date/Time In Seconds() -> (seconds since 1Jan1904=w132:timestamp)
              n28 = Subtract(x=w132, y=w128) -> (x-y=w130:dbl)
              n29 = Set File Position(refnum=w118, from (0:start)=enum16{"start", "end", "current"}."end", error in=w126) -> (refnum out=w136:refnum<file>, error out=w137:errorcluster)  [unwired: 1 in]
              n30 = case "have written headers?" shown="True" w117 {
                selector: w117 -> [_ w145]
                tunnel: [w143 w147] -> w134
                tunnel: w137 -> [w144 w147]
                tunnel: w136 -> [w141 w146]
                tunnel: [w142 w146] -> w135
                tunnel: w127 -> [w140 _]
                tunnel: [TRUE w145] -> w116
                frame False {
                  n31 = call "Write Headers.vi"("error in (no error)"=w144, "data"=w140, "Byte Stream File in"=w141) -> ("error out"=w143:errorcluster, "Byte Stream File out"=w142:refnum<file>)  [unwired: 7 in]
                }
                frame True {
                }
              }
              n32 = Get Date/Time String(seconds (now)=w130, want seconds? (F)=TRUE) -> (time string=w131:string)  [unwired: 1 in, 1 out]
              n33 = call "Data to CSV Line.vi"("error in (no error)"=w134, "Elapsed Time"=w131, "Array"=w127) -> ("error out"=w133:errorcluster, "Spreadsheet String"=w122:string[])  [unwired: 7 in]
              n34 = Build Array (concatenate)(w122, w125) -> (w121:string[])
              n35 = Array To Spreadsheet String(delimiter (Tab)=",", array=w121, 3:"%f" ("format string")) -> (spreadsheet string=w119:string)
              n36 = Write to Text File(file (use dialog)=w135, text=w119, error in=w133) -> (refnum out=w115:refnum<file>, error out=w120:errorcluster)  [unwired: 1 in, 1 out]
              n37 = in-place-cluster #1("CSV refnum"=w115, "Have written headers?"=w116) -> (w100:T66)
            }
          }
          frame "Stop" {
            n38 = Unbundle By Name(w149) -> ("CSV refnum"=w157:refnum<file>)
            n39 = Close File(refnum=w157, error in=w158) -> (error out=w152:errorcluster)  [unwired: 1 out]
            n40 = in-place {
              # "close the CSV file"
              n41 = in-place-cluster #2(w149) -> ()  [unwired: 1 out]
              n42 = in-place-cluster #2("CSV refnum"=refnum<file> refnum) -> (w148:T66)
            }
            n43 = call <vilib>:"Clear Errors.vi"("error in (no error)"=w152, "specific error code to clear (0: all)"=1) -> ("error out"=w151:errorcluster)  [unwired: 4 in, 1 out]
            n44 = call "Write to Log File.vi"("error in"=w151, "text"="Data Log: Stopped") -> ()  [unwired: 9 in, 1 out]
          }
          frame "Exit" {
            n45 = call-poly "Enqueue Message.vi"("error in (no error)"=w167, "Message"="Exit", "Message Queue"=w168) -> ("error out"=w163:errorcluster)  [unwired: 7 in, 1 out]
            n46 = flat-sequence {
              tunnel: w165 -> [w177]
              tunnel: w163 -> [w176]
              tunnel: [w175] -> w161
              tunnel: [w179] -> w162
              tunnel: w161 -> [w179]
              tunnel: w164 -> [w183]
              tunnel: w162 -> [w182]
              tunnel: [w181] -> w160
              frame #0 {
                n47 = call-poly "Enqueue Message.vi"("error in (no error)"=w176, "Message"="Exit", "Message Queue"=w177) -> ("error out"=w175:errorcluster)  [unwired: 7 in, 1 out]
              }
              frame #1 {
                n48 = Wait (ms)(milliseconds to wait=u32 100) -> ()  [unwired: 1 out]
              }
              frame #2 {
                n49 = call-poly "Enqueue Message.vi"("error in (no error)"=w182, "Message"="Exit", "Message Queue"=w183) -> ("error out"=w181:errorcluster)  [unwired: 7 in, 1 out]
              }
            }
            n50 = call "Write to Log File.vi"("error in"=w160, "text"="Data Log: Exited") -> ()  [unwired: 9 in, 1 out]
          }
        }
      }
    }
    frame Error {
    }
  }
  "error out" <- w9
  n51 = while "Note Dialog Loop" {
    tunnel: w8 -> [w192]
    tunnel: w5 -> [w191]
    tunnel: w4 -> [w190]
    stop <- w188 stop-if-true
    n52 = call "Dequeue Message.vi"("error in (no error)"=w190, "Message Queue"=w191) -> ("error out"=w187:errorcluster, "Message"=w189:string)  [unwired: 6 in, 2 out]
    n53 = case shown="\"Open Note Dialog\"" w189 {
      tunnel: w192 -> [_ w197 _]
      tunnel: [_ _ TRUE] -> w188
      tunnel: w187 -> [_ w196 _]
      frame Default {
      }
      frame "Open Note Dialog" {
        n54 = call "Note Dialog.vi"("error in (no error)"=w196) -> ("error out"=w193:errorcluster, "Note"=w194:string, "OK"=w195:bool)  [unwired: 8 in]
        n55 = case "OK?" shown="True" w195 {
          tunnel: w194 -> [_ w207]
          tunnel: w197 -> [_ w202]
          tunnel: w193 -> [_ w200]
          frame False {
          }
          frame True {
            # "Remove \",\" to avoid issues in excel"
            n56 = Search and Replace String(replace all?=TRUE ("replace all? (F)"), input string=w207, search string=",", replace string=" " ("replace string (\"\")"), error in=w200) -> (result string=w203:string, error out=w198:errorcluster)  [unwired: 3 in, 2 out]
            n57 = call-poly "Enqueue Message.vi"("Message Data"=w203, "Message"="File Note", "Message Queue"=w202) -> ()  [unwired: 7 in, 2 out]
            n58 = call "Write to Log File.vi"("error in"=w198, "text"="Data Log: Note Added") -> ()  [unwired: 9 in, 1 out]
          }
        }
      }
      frame "Exit" {
      }
    }
  }
  n59 = Release Queue(queue=w1) -> ()  [unwired: 2 in, 3 out]
